vi "worksheet gridlines.vi"(8 "error in (no error)":errorcluster, 10 "option":u8, 11 "worksheet":u32) -> (0 "error out":errorcluster)   [LabVIEW 2015, in "xlsxwriter.lvlib"]
doc: "void worksheet_gridlines(lxw_worksheet worksheet, uint8_t option);"
uses:
  xlsxwriter.lvlib
  xlsxwriter.dll
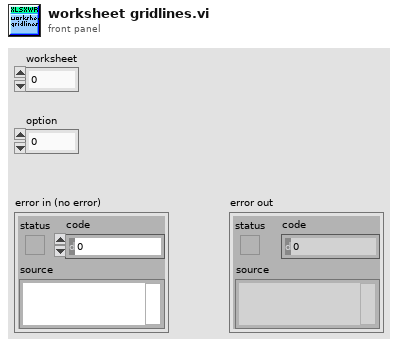
[diagram p1: front panel]
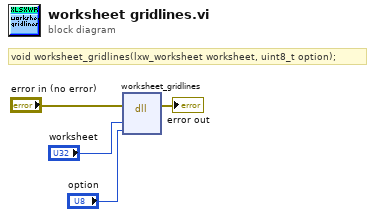
[diagram p0: block diagram]
diagram:
  # "void worksheet_gridlines(lxw_worksheet worksheet, uint8_t option);"
  n1 = dll-call lib="C:/Users/WDAGUtilityAccount/Desktop/lv_vis_added_cell/xlsxwriter.*" fn="worksheet_gridlines"(error in="error in (no error)", "worksheet"="worksheet", "option"="option") -> (error out=→"error out":errorcluster)  [unwired: 5 in, 1 out]
